vi "Cel2Farh.vi"() -> ()   [LabVIEW 2020]
panel:
  in  "stop":bool
  out "Temp in F":dbl
  in  "Temp in C":dbl
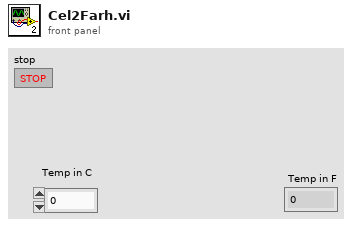
[diagram p1: front panel]
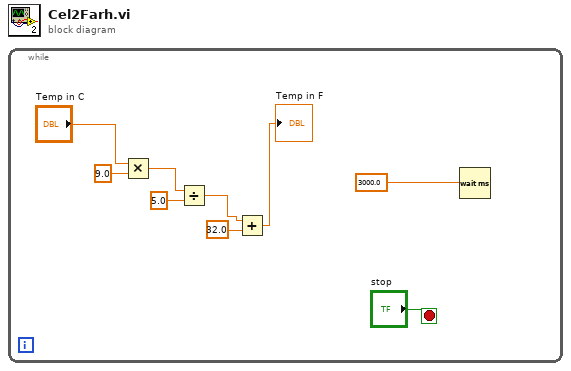
[diagram p0: block diagram]
diagram:
  n1 = while {
    stop <- "stop" stop-if-true
    n2 = Multiply(x="Temp in C", y=9.0) -> (x*y=w7:dbl)
    n3 = Divide(x=w7, y=5.0) -> (x/y=w5:dbl)
    n4 = Add(x=w5, y=32.0 ("x+y")) -> (x+y=→"Temp in F":dbl)
    n5 = Wait (ms)(milliseconds to wait=3000.0 ("x+y")) -> ()  [unwired: 1 out]
  }
